vi "rollback_transaction.vi"(0 "DB Session ID":i32, 11 "error in (no error)":errorcluster) -> (4 "DB Session ID out":i32, 15 "error out":errorcluster)   [LabVIEW 2017, in "Database.lvlib"]
uses:
  Database.lvlib
  bin/Database.dll
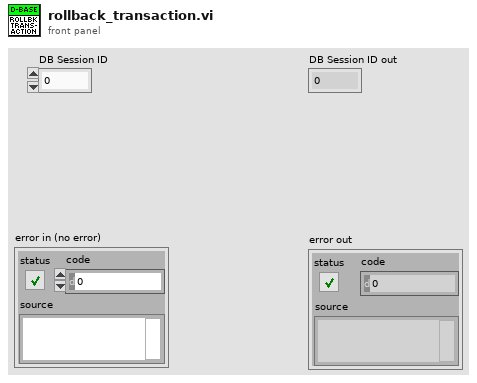
[diagram p1: front panel]
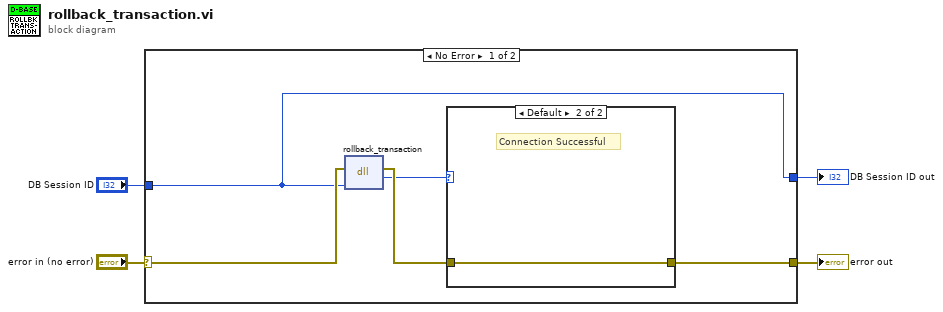
[diagram p0: block diagram]
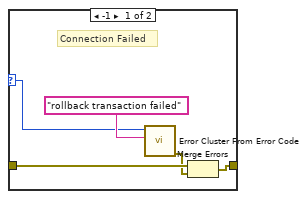
[diagram p2: hidden frame]
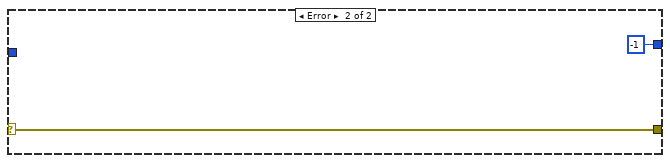
[diagram p3: hidden frame]
diagram:
  n1 = case shown="No Error" "error in (no error)" {
    selector: "error in (no error)" -> [w9 w17]
    tunnel: [w7 w17] -> w3
    tunnel: [w5 -1 ("return type")] -> w2
    tunnel: "DB Session ID" -> [w5 _]
    frame No Error {
      n2 = dll-call lib="C:/Users/Caleb/Desktop/nebraska-silicon-lab/pixel-gantry-extra/LV/bin/Database.dll" fn="rollback_transaction"(error in=w9, "conn_id"=w5) -> (error out=w8:errorcluster, "return type"=w6:i32)  [unwired: 3 in, 1 out]
      n3 = case shown="Default" w6 {
        selector: w6 -> [w10 _]
        tunnel: w8 -> [w14 w15]
        tunnel: [w13 w15] -> w7
        frame -1 {
          # "Connection Failed"
          n4 = call <vilib>:"Error Cluster From Error Code.vi"("error message (\"\")"="rollback transaction failed" ("error message (\"\")"), "error code (0)"=w10) -> ("error out"=w12:errorcluster)  [unwired: 7 in]
          n5 = Merge Errors(w14, w12) -> (w13:errorcluster)
        }
        frame Default {
          # "Connection Successful"
        }
      }
    }
    frame Error {
    }
  }
  "error out" <- w3
  "DB Session ID out" <- w2
